vi "MT Measure PSK Quadrature Impairments.vi"(0 "recovered complex waveform":T7={"t0"=0.0, "dt"=1.0, "Y"=[]} {"Y" format="%.3f"; "dt" format="%^.2e"; "t0" format="%.4f"}, 1 "PSK system parameters":T3={"samples per symbol (16)"=16, "symbol map"=[], "differential PSK"=enum."disable", "PSK type"=0} {"PSK type" items=["normal", "shifted", "offset"]; "symbol map" format="%.3f"}, 5 "input bit stream":i8[](array[numeric]), 7 "impairment measurement window":T4={"start index (symbols)"=0, "width (symbols) (-1: all)"=-1}, 11 "error in (no error)":errorcluster, 12 "impairment definition":enum16{"Vertical Shear", "Axis Shear"}(ring), 13 "reset? (T)":bool=TRUE) -> (2 "magnitude error":T2 {"individual symbol measurements (%)" format="%.2f"; "peak measurement (%)" format="%.2f"; "RMS measurement (%)" format="%.2f"}, 3 "DC offset measurements":T5 {"origin offset (dB)" format="%.2f"; "Q (%)" format="%.2f"; "I (%)" format="%.2f"}, 4 "IQ gain imbalance (dB)":dbl format="%.2f", 6 "phase error":T6 {"individual symbol measurements (deg)" format="%.2f"; "peak measurement (deg)" format="%.2f"; "RMS measurement (deg)" format="%.2f"}, 8 "EVM":T2 {"individual symbol measurements (%)" format="%.2f"; "peak measurement (%)" format="%.2f"; "RMS measurement (%)" format="%.2f"}, 10 "modulation error ratio (dB)":dbl format="%.2f", 14 "quadrature skew (deg)":dbl format="%.2f", 15 "error out":errorcluster)   [LabVIEW 2020, in "niDMT.lvlib"]
doc: "This polymorphic instance calculates and reports PSK quadrature impairments on a symbol-by-symbol basis at the symbol timing."
uses:
  <vilib>/addons/Modulation/niDMT.lvlib
  <vilib>/addons/Modulation/Analog/controls/Complex Data Waveform.ctl
  <vilib>/addons/Modulation/Digital/Support/Controls/Offset PSK System Parameters.ctl
  <vilib>/addons/Modulation/niAMT.lvlib
panel:
  out "Offset EVM":T1
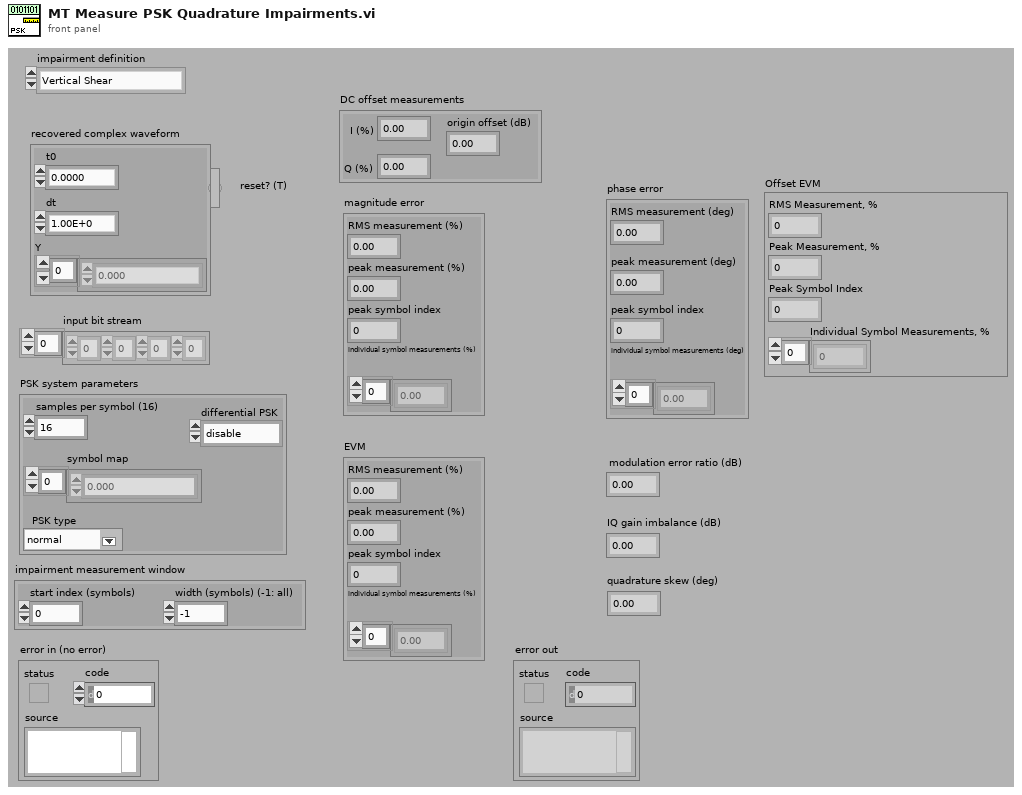
[diagram p1: front panel]
types:
  T1 = cluster{"RMS Measurement, %":dbl, "Peak Measurement, %":dbl, "Peak Symbol Index":i32, "Individual Symbol Measurements, %":dbl[]}
  T2 = cluster{"RMS measurement (%)":dbl, "peak measurement (%)":dbl, "peak symbol index":i32, "individual symbol measurements (%)":dbl[]}
  T3 = cluster{"samples per symbol (16)":i32, "symbol map":cdb[], "differential PSK":enum16{"disable", "enable"}, "PSK type":u16}
  T4 = cluster{"start index (symbols)":i32, "width (symbols) (-1: all)":i32}
  T5 = cluster{"I (%)":dbl, "Q (%)":dbl, "origin offset (dB)":dbl}
  T6 = cluster{"RMS measurement (deg)":dbl, "peak measurement (deg)":dbl, "peak symbol index":i32, "individual symbol measurements (deg)":dbl[]}
  T7 = typedef "niAMT.lvlib/Complex Data Waveform.ctl" = cluster{"t0":dbl, "dt":dbl, "Y":cdb[]}
  T8 = enum16{"FSK", "PSK", "QAM", "MSK", "PAM", "ASK", "CPM"}
  T9 = cluster{"I, %":dbl, "Q, %":dbl, "Origin Offset, dB":dbl}
  T10 = typedef "niDMT.lvlib/Offset PSK System Parameters.ctl" = cluster{"samples per symbol (16)":i32, "symbol map":cdb[], "differential Offset PSK":enum16{"disable", "enable"}}
  T11 = cluster{"RMS Measurement, deg":dbl, "Peak Measurement, deg":dbl, "Peak Symbol Index":i32, "Individual Symbol Measurements, deg":dbl[]}
  T12 = cluster{"RMS measurement, %":dbl, "peak measurement, %":dbl, "peak symbol index":i32, "individual symbol\n measurements, %":dbl[]}
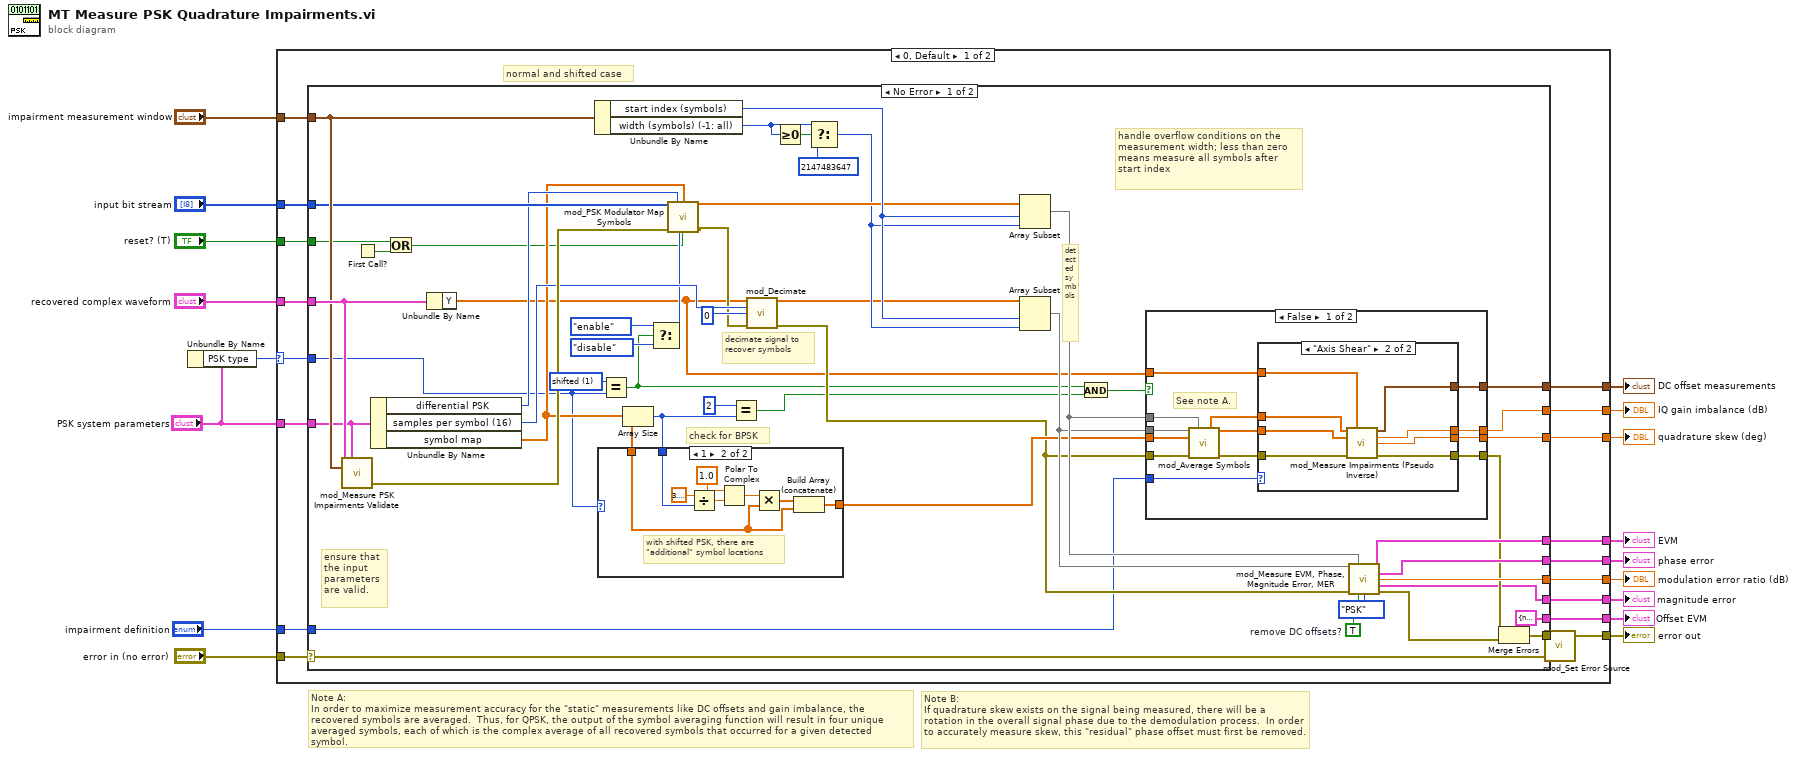
[diagram p0: block diagram]
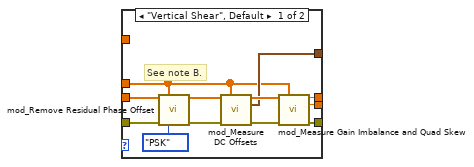
[diagram p2: hidden frame]
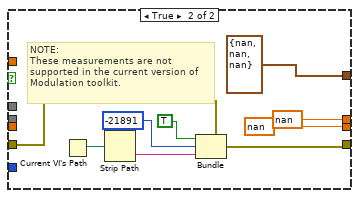
[diagram p3: hidden frame]
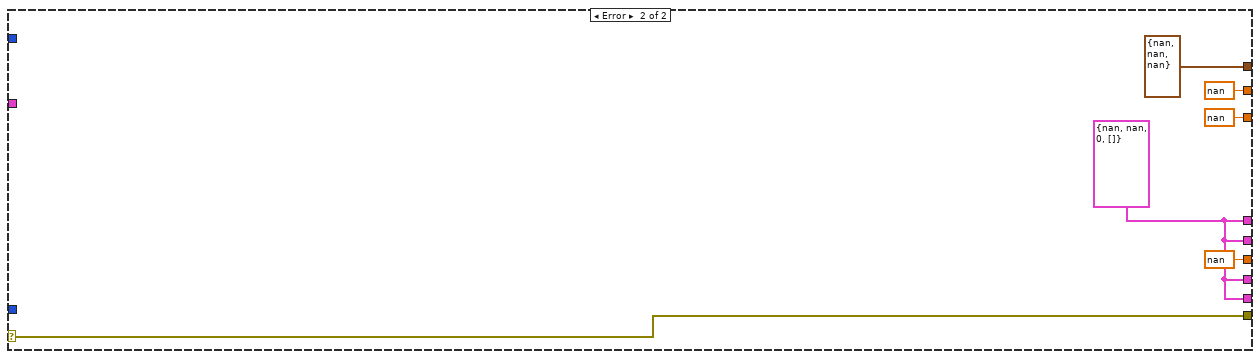
[diagram p5: hidden frame]
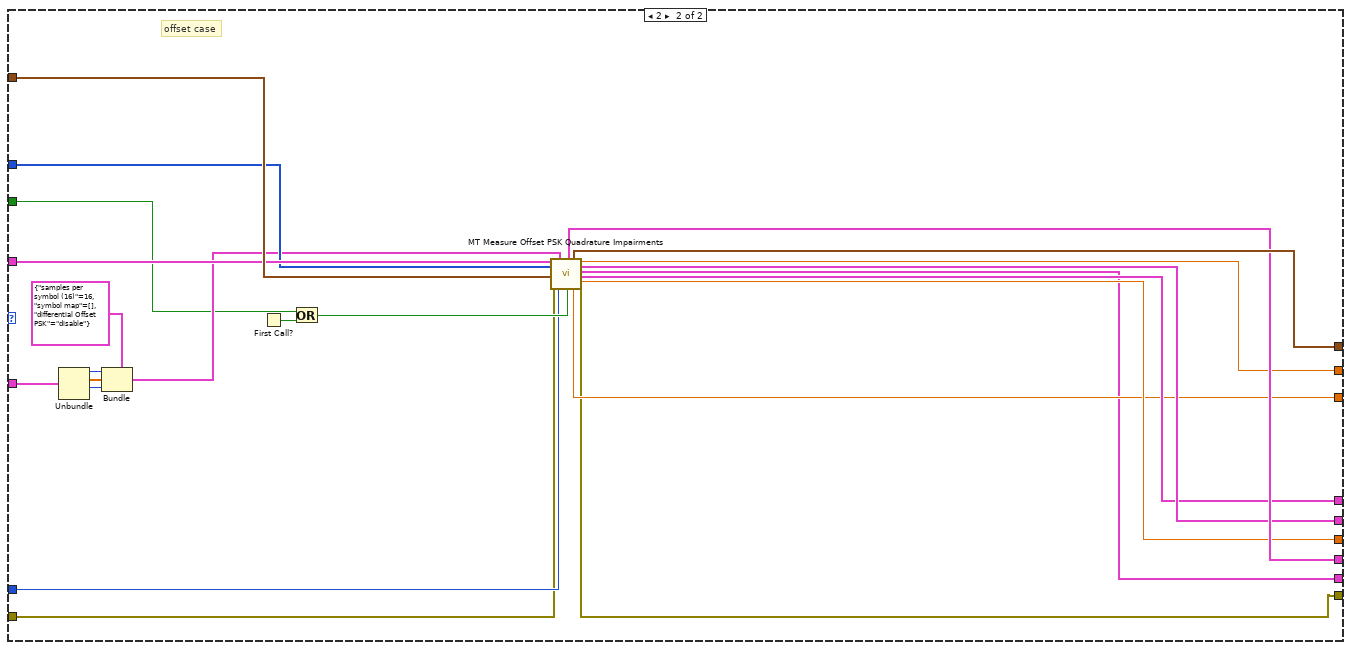
[diagram p6: hidden frame]
diagram:
  # "Note A:\nIn order to maximize measurement accuracy for the \"static\" measurements like DC offsets and gain imbalance, the recovered symbols are averaged.  Thus, for QPSK, the output of the symbol averaging function will result in four unique averaged symbols, each of which is the complex average of all recovered symbols that occurred for a given detected symbol."
  # "Note B:\nIf quadrature skew exists on the signal being measured, there will be a rotation in the overall signal phase due to the demodulation process.  In order to accurately measure skew, this \"residual\" phase offset must first be removed."
  n1 = Unbundle By Name("PSK system parameters") -> ("PSK type"=w4:u16)
  n2 = case shown="0, Default" w4 {
    selector: w4 -> [w20 _]
    tunnel: "error in (no error)" -> [w34 w144]
    tunnel: "recovered complex waveform" -> [w33 w164]
    tunnel: [w32 w154] -> w15
    tunnel: [w31 w153] -> w14
    tunnel: [w30 w155] -> w13
    tunnel: [w29 w143] -> w2
    tunnel: "input bit stream" -> [w28 w163]
    tunnel: "impairment measurement window" -> [w27 w165]
    tunnel: [w26 w152] -> w10
    tunnel: [w25 w151] -> w9
    tunnel: [w24 w157] -> w8
    tunnel: "reset? (T)" -> [w23 w149]
    tunnel: [w22 w156] -> w6
    tunnel: "PSK system parameters" -> [w21 w162]
    tunnel: "impairment definition" -> [w19 w146]
    tunnel: [w18 w145] -> w1
    frame 0, Default {
      # "normal and shifted case"
      n3 = case shown="No Error" w34 {
        selector: w34 -> [w76 w142]
        tunnel: w33 -> [w83 _]
        tunnel: [w78 T9 {"I, %"=nan, "Q, %"=nan, "Origin Offset, dB"=nan} ("DC Offset Measurements")] -> w24
        tunnel: [w80 w138] -> w32
        tunnel: [w85 w138] -> w31
        tunnel: [w72 nan ("IQ Gain Imbalance, dB")] -> w30
        tunnel: [w75 w142] -> w29
        tunnel: w28 -> [w69 _]
        tunnel: w27 -> [w81 _]
        tunnel: [w79 nan ("Modulation Error Ratio, dB")] -> w26
        tunnel: [w73 nan ("Quadrature Skew, deg")] -> w25
        tunnel: w21 -> [w71 _]
        tunnel: w23 -> [w46 _]
        tunnel: [w54 w138] -> w22
        tunnel: w20 -> [w40 _]
        tunnel: w19 -> [w39 _]
        tunnel: [T1 {"RMS Measurement, %"=nan, "Peak Measurement, %"=nan, "Peak Symbol Index"=0, "Individual Symbol Measurements, %"=[]} ("EVM") w138] -> w18
        frame No Error {
          w42 = u16 1 items=["normal", "shifted", "offset"] ("PSK type")
          w61 = TRUE  # remove DC offsets?
          # "check for BPSK"
          # "decimate signal to recover symbols"
          # "ensure that the input parameters are valid."
          # "detected symbols"
          # "handle overflow conditions on the\nmeasurement width; less than zero\nmeans measure all symbols after\nstart index"
          n4 = call <vilib>:"mod_Measure PSK Impairments Validate.vi"("Input Complex Waveform"=w83, "PSK System Parameters"=w71, "Impairment Measurement Window"=w81) -> ("error out"=w65:errorcluster)  [unwired: 12 out]
          n5 = First Call?() -> (First Call?: T/F=w45:bool)
          n6 = Unbundle By Name(w71) -> ("differential PSK"=w68:enum16{"disable", "enable"}, "samples per symbol (16)"=w63:i32, "symbol map"=w49:cdb[])
          n7 = Or(x=w46, y=w45) -> (x .or. y?=w44:bool)
          n8 = Unbundle By Name(w83) -> ("Y"=w37:cdb[])
          n9 = Unbundle By Name(w81) -> ("start index (symbols)"=w82:i32, "width (symbols) (-1: all)"=w55:i32)
          n10 = Equal?(x=w42, y=w40) -> (x = y?=w50:bool)
          n11 = Array Size(array=w49) -> (size(s)=w41:i32)
          n12 = case shown="1" w40 {
            tunnel: [w128 w132] -> w62
            tunnel: w49 -> [w128 w130]
            tunnel: w41 -> [_ w129]
            frame 0, Default {
              # "normal psk"
            }
            frame 1 {
              # "with shifted PSK, there are \"additional\" symbol locations"
              n13 = Divide(x=3.141592653589793, y=w129) -> (x/y=w135:dbl)
              n14 = Polar To Complex(1:w135, 2:1.0) -> (0:w133:cdb)
              n15 = Multiply(x=w133, y=w130) -> (x*y=w131:cdb[])
              n16 = Build Array (concatenate)(w131, w130) -> (w132:cdb[])
            }
          }
          n17 = Select(t=enum16{"disable", "enable"}."enable" ("Shifted PSK Enable (disable)"), s=w50, f=enum16{"disable", "enable"}."disable" ("Shifted PSK Enable (disable)")) -> (s? t:f=w51:enum16{"disable", "enable"})
          n18 = call <vilib>:"mod_PSK Modulator Map Symbols.vi"("Input Bit Stream"=w69, "Differential PSK Enable (disable)"=w68, "Symbol Map"=w49, "error in (no error)"=w65, "Shifted PSK Enable (disable)"=w51, "Reset? (T)"=w44) -> ("Symbols"=w64:cdb[], "error out"=w60:errorcluster)  [unwired: 1 in, 7 out]
          n19 = Equal?(x=2 ("y"), y=w41) -> (x = y?=w48:bool)
          n20 = call <vilib>:"mod_Decimate.vi"("Signal In"=w37, "Samples Per Symbol (16)"=w63, "Offset"=0, "error in (no error)"=w60) -> ("Signal Out"=w36:cdb[], "error out"=w59:errorcluster)  [unwired: 1 in, 9 out]
          n21 = Greater Or Equal To 0?(x=w55) -> (x >= 0?=w58:bool)
          n22 = Select(t=w55, s=w58, f=2147483647) -> (s? t:f=w56:i32)
          n23 = Array Subset(array=w64, index=w82, length=w56) -> (w67:cdb[])
          n24 = Array Subset(array=w36, index=w82, length=w56) -> (w66:cdb[])
          n25 = And(x=w50, y=w48) -> (x .and. y?=w47:bool)
          n26 = case shown="False" w47 {
            tunnel: [w98 T9 {"I, %"=nan, "Q, %"=nan, "Origin Offset, dB"=nan} ("DC Offset Measurements")] -> w78
            tunnel: [w97 w119] -> w74
            tunnel: [w96 nan ("Quadrature Skew, deg")] -> w73
            tunnel: [w95 nan ("IQ Gain Imbalance, dB")] -> w72
            tunnel: w67 -> [w91 _]
            tunnel: w66 -> [w87 _]
            tunnel: w62 -> [w90 _]
            tunnel: w59 -> [w89 w124]
            tunnel: w39 -> [w88 _]
            tunnel: w37 -> [w86 _]
            frame False {
              # "See note A."
              n27 = call <vilib>:"mod_Average Symbols.vi"("Recovered Symbols"=w87, "Detected Symbols"=w91, "Symbol Map"=w90, "error in (no error)"=w89) -> ("Grouped Detected Symbols"=w93:cdb[], "Averaged Symbols"=w92:cdb[], "error out"=w94:errorcluster)  [unwired: 9 out]
              n28 = case shown="\"Axis Shear\"" w88 {
                tunnel: [w108 w115] -> w98
                tunnel: [w107 w112] -> w97
                tunnel: [w106 w113] -> w96
                tunnel: [w105 w114] -> w95
                tunnel: w94 -> [w104 w117]
                tunnel: w93 -> [w102 w118]
                tunnel: w92 -> [w101 w116]
                tunnel: w86 -> [_ w111]
                frame "Vertical Shear", Default {
                  # "See note B."
                  n29 = call <vilib>:"mod_Remove Residual Phase Offset.vi"("Averaged Symbols In"=w101, "Grouped Detected Symbols"=w102, "error in (no error)"=w104, "Modulation Type"=T8."PSK") -> ("Averaged Symbols Out"=w100:cdb[], "error out"=w103:errorcluster)  [unwired: 10 out]
                  n30 = call <vilib>:"mod_Measure DC Offsets.vi"("Averaged Symbols"=w100, "Grouped Detected Symbols"=w102, "error in (no error)"=w103) -> ("Corrected Symbols"=w109:cdb[], "DC Offset Measurements"=w108:T9, "error out"=w110:errorcluster)  [unwired: 1 in, 9 out]
                  n31 = call <vilib>:"mod_Measure Gain Imbalance and Quad Skew.vi"("Corrected Symbols"=w109, "Grouped Detected Symbols"=w102, "error in (no error)"=w110) -> ("IQ Gain Imbalance, dB"=w105:dbl, "Quadrature Skew, deg"=w106:dbl, "error out"=w107:errorcluster)  [unwired: 1 in, 9 out]
                }
                frame "Axis Shear" {
                  n32 = call <vilib>:"mod_Measure Impairments (Pseudo Inverse).vi"("Grouped detected symbols"=w118, "Recovered Complex Waveform"=w111, "Averaged symbols"=w116, "error in (no error)"=w117) -> ("DC Offset Measurements"=w115:T9, "IQ gain imbalance (dB)"=w114:dbl, "quadrature skew (deg)"=w113:dbl, "error out"=w112:errorcluster)  [unwired: 8 out]
                }
              }
            }
            frame True {
              # "NOTE:\nThese measurements are not\nsupported in the current version of\nModulation toolkit."
              n33 = Current VI's Path() -> (path=w121:path)
              n34 = Strip Path(path=w121) -> (name=w120:string)  [unwired: 1 out]
              n35 = Bundle(cluster=w124, "status"=TRUE, "code"=-21891, "source"=w120) -> (w119:errorcluster)
            }
          }
          n36 = call <vilib>:"mod_Measure EVM, Phase, Magnitude Error, MER.vi"("Recovered Signal"=w66, "Detected Signal"=w67, "error in (no error)"=w59, "remove DC offsets? (T)"=w61, "Modulation Type"=T8."PSK") -> ("EVM"=w85:T1, "Phase Error"=w80:T11, "Modulation Error Ratio, dB"=w79:dbl, "magnitude error"=w54:T1, "error out"=w84:errorcluster)  [unwired: 1 in, 5 out]
          n37 = Merge Errors(w74, w84) -> (w77:errorcluster)
          n38 = call <vilib>:"mod_Set Error Source.vi"("initial error in (no error)"=w76, "final error in (no error)"=w77) -> ("error out"=w75:errorcluster)  [unwired: 3 out]
        }
        frame Error {
          w138 = T1 {"RMS Measurement, %"=nan, "Peak Measurement, %"=nan, "Peak Symbol Index"=0, "Individual Symbol Measurements, %"=[]} ("EVM")
        }
      }
    }
    frame 2 {
      # "offset case"
      n39 = Unbundle(w162) -> ("samples per symbol (16)"=w161:i32, "symbol map"=w160:cdb[], "differential PSK"=w159:enum16{"disable", "enable"})  [unwired: 1 out]
      n40 = Bundle(cluster=T10 {"samples per symbol (16)"=16, "symbol map"=[], "differential Offset PSK"=enum."disable"} ("Offset PSK System Parameters"), "samples per symbol (16)"=w161, "symbol map"=w160, "differential Offset PSK"=w159) -> (w158:T10)
      n41 = First Call?() -> (First Call?: T/F=w150:bool)
      n42 = Or(x=w149, y=w150) -> (x .or. y?=w148:bool)
      n43 = call <vilib>:"MT Measure Offset PSK Quadrature Impairments.vi"("recovered complex waveform"=w164, "input bit stream"=w163, "impairment measurement window"=w165, "error in (no error)"=w144, "Offset PSK System Parameters"=w158, "impairment definition"=w146, "reset? (T)"=w148) -> ("magnitude error"=w156:T2, "DC offset measurements"=w157:T5, "quadrature skew (deg)"=w151:dbl, "IQ gain imbalance (dB)"=w155:dbl, "phase error"=w154:T6, "Offset EVM"=w145:T2, "EVM"=w153:T12, "modulation error ratio (dB)"=w152:dbl, "error out"=w143:errorcluster)  [unwired: 4 in]
    }
  }
  "error out" <- w2
  "IQ gain imbalance (dB)" <- w13
  "quadrature skew (deg)" <- w9
  "phase error" <- w15
  "EVM" <- w14
  "modulation error ratio (dB)" <- w10
  "DC offset measurements" <- w8
  "magnitude error" <- w6
  "Offset EVM" <- w1
